vi "Maxi Gauge-RW Calibration factor.vi"(0 "VISA-Ressource in":refnum<visa-resource-name>, 1 "W/R":bool, 5 "Node address":i8=-1 min=-1 max=31 step=1, 7 "Sensor Nr.:":i32(ring) items=["sensor 1", "sensor 2", "sensor 3", "sensor 4", "sensor 5", "sensor 6"], 9 "Set Calibration factor":dbl=1.0 min=0.1 max=9.999 step=0.001 format="%.3f", 11 "Fehler (Eingang)":errorcluster) -> (4 "VISA-Ressource out":refnum<visa-resource-name>, 10 "Get Calibration factor":dbl=0.000753 format="%.3f", 15 "Fehler (Ausgang)":errorcluster)   [LabVIEW 2012, in "Maxi Gauge.lvlib"]
uses:
  Maxi Gauge.lvlib
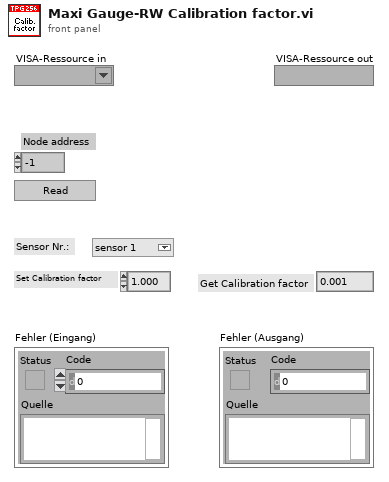
[diagram p1: front panel]
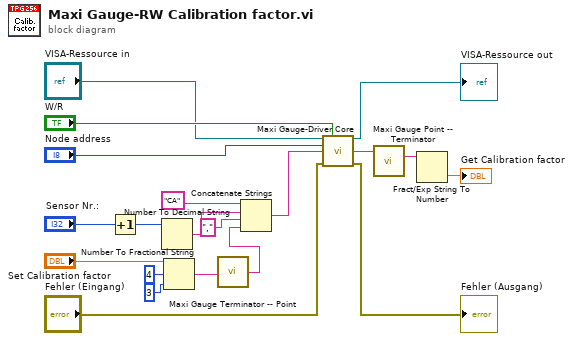
[diagram p0: block diagram]
diagram:
  n1 = Increment(x="Sensor Nr.:") -> (x+1=w19:i32)
  n2 = Number To Decimal String(number=w19) -> (decimal integer string=w12:string)  [unwired: 1 in]
  n3 = Number To Fractional String(number="Set Calibration factor", width (-)=i16 4, precision (6)=i16 3) -> (F-format string=w9:string)  [unwired: 1 in]
  n4 = call "Maxi Gauge Terminator -- Point.vi"("Eingangstring"=w9) -> ("Ausgangstring"=w8:string)
  n5 = Concatenate Strings("CA", w12, "," ("Ausgangstring"), w8) -> (w5:string)
  n6 = call "Maxi Gauge-Driver Core.vi"("VISA-Ressource in"="VISA-Ressource in", "Write/Read"="W/R", "Node address"="Node address", "Command"=w5, "Fehler (Eingang)"="Fehler (Eingang)") -> ("VISA-Ressource out"=→"VISA-Ressource out":refnum<visa-resource-name>, "String Out"=w14:string, "Fehler (Ausgang)"=→"Fehler (Ausgang)":errorcluster)  [unwired: 8 in]
  n7 = call "Maxi Gauge Point -- Terminator.vi"("Eingangstring"=w14) -> ("Ausgangstring"=w6:string)
  n8 = Fract/Exp String To Number(string=w6) -> (number=→"Get Calibration factor":dbl)  [unwired: 3 in, 1 out]
